vi "BiaxXsig process (16chan).vi"(0 "voltage data":sgl[](array[numeric]) format="%.2f", 3 "Numeric":i32=4, 7 "error in (no error)":errorcluster) -> (8 "signal to file (Volt)":sgl[](array[numeric]) format="%.2f", 9 "AUX8":dbl format="%.2f", 10 "AUX9":dbl format="%.2f", 11 "Hor LVDT":dbl format="%.2f", 12 "AUX7":dbl format="%.2f", 13 "AUX6":dbl format="%.2f", 14 "AUX5":dbl format="%.2f", 15 "error out":errorcluster, 16 "AUX12":dbl format="%.2f", 17 "AUX4":dbl format="%.2f", 18 "AUX11":dbl format="%.2f", 19 "AUX10":dbl format="%.2f", 20 "Hor Load":dbl format="%.2f", 21 "Vert Load":dbl format="%.2f", 23 "Ver LVDT":dbl format="%.2f", 24 "AUX1":dbl format="%.2f", 25 "AUX2":dbl format="%.2f", 27 "AUX3":dbl format="%.2f")   [LabVIEW 2013]
doc: "This vi accepts the raw voltage data from the following channels: \nCh 0 = Conf. Press. Amp. (0-5)\nCh 1 = Fluid Press. Amp (0-5)\nCh 2 = Temp. Amp (0-1.25 V)\nCh 3 = Displacement Transducer (-2.5 to +2.5 Volt)The data is acquired and processed one point at a time (a non-buffered acquisition). \nCh 4 = Load cell after amplification. 12600 lbsf/volt \n\nThe voltage data array contains the data that the example VI just retrieved from the buffer, one sample per channel. It is a one-dimensional array, indexed by channel.\n\nThe processed data array is returned to the example VI to be displayed.\n\nError in is a cluster that indicates if an error has occurred. If so, this VI does not try to process the data, it just returns the voltage data and error unchanged. If an error occurs in your data processing, you should set the following values in the error out cluster:\n\n (bool) status: TRUE.\n\n (i32) code: the error code associated with an error.\n A value of 0 means no error, a negative value is an error,\n and a positive value is a warning.\n\n (string) source: an indication of where the \n error occurred, usually the name of the VI."
panel:
  # "Sig. Eng. Units"
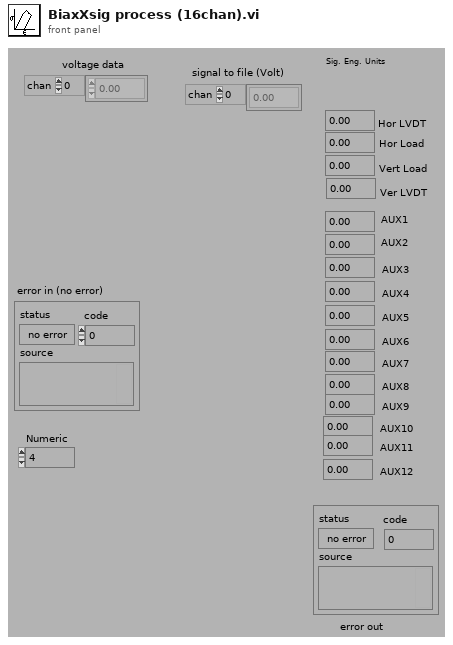
[diagram p1: front panel]
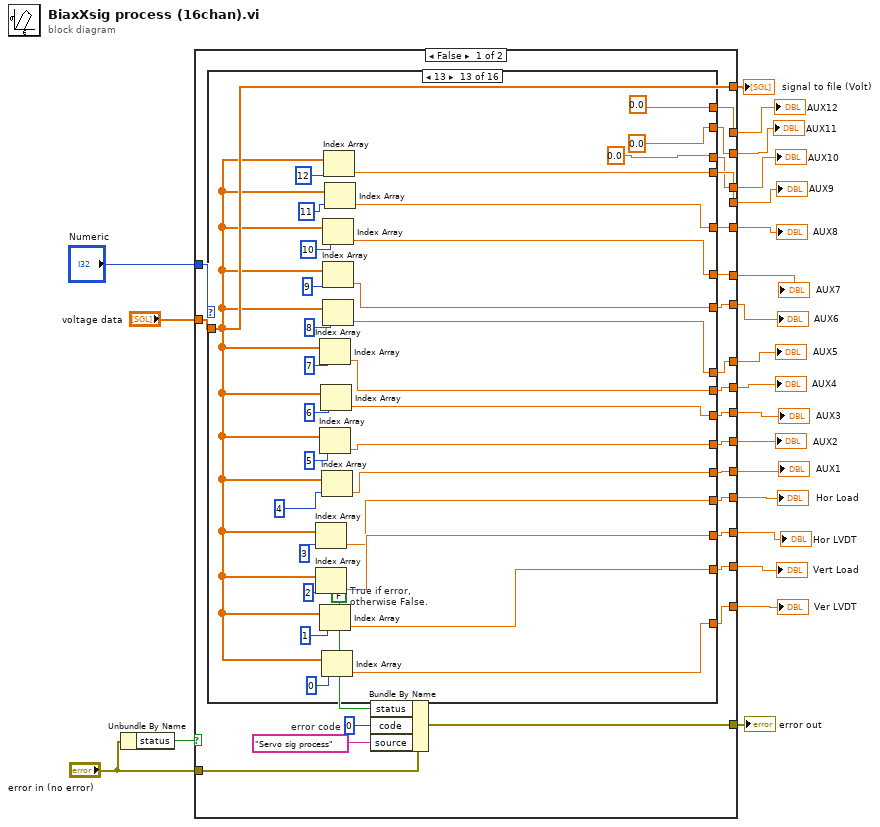
[diagram p0: block diagram]
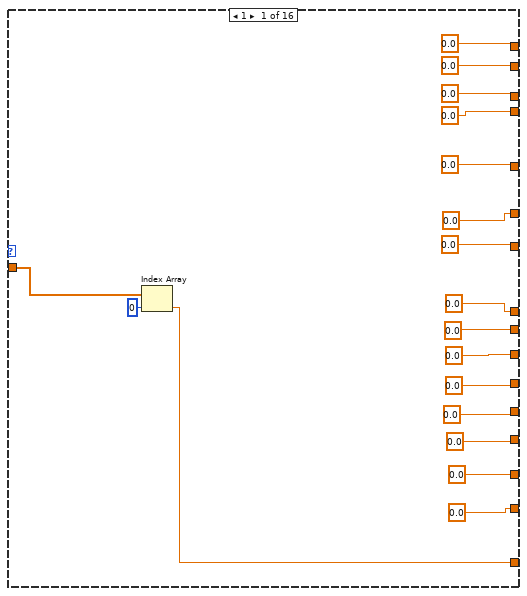
[diagram p2: hidden frame]
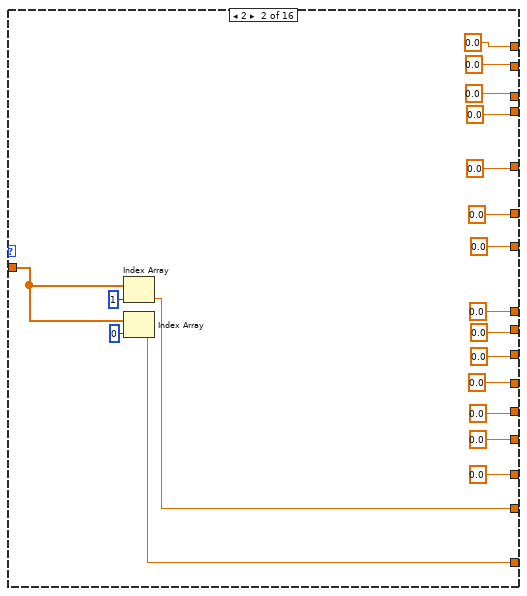
[diagram p3: hidden frame]
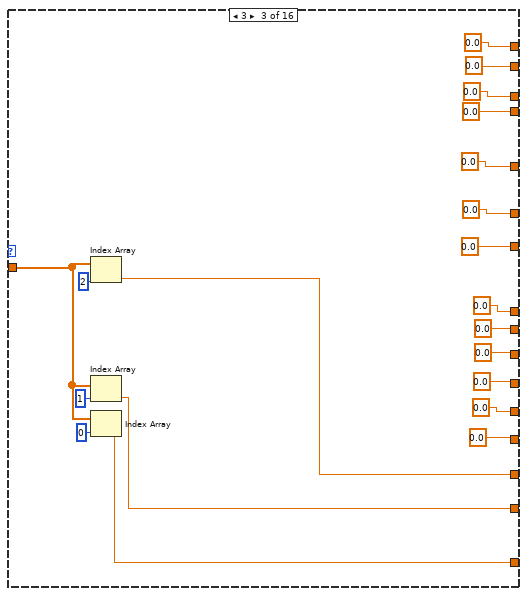
[diagram p4: hidden frame]
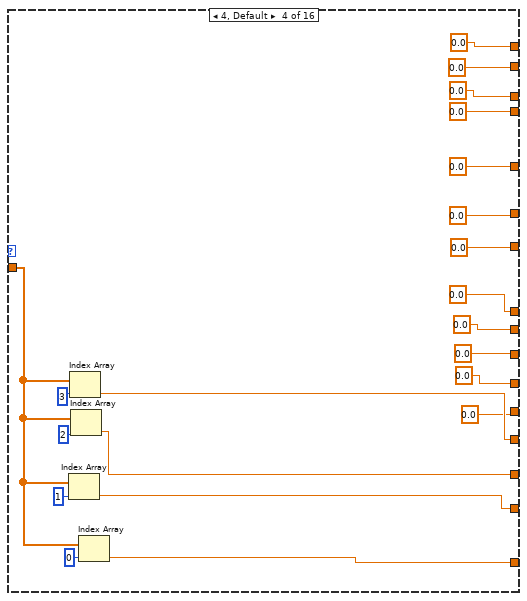
[diagram p5: hidden frame]
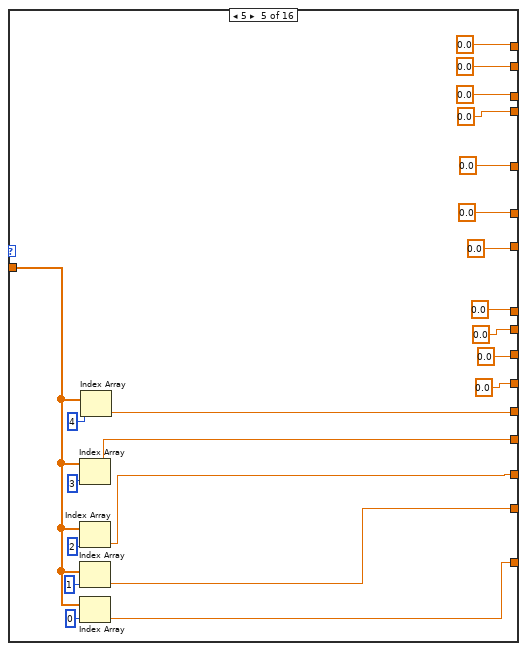
[diagram p6: hidden frame]
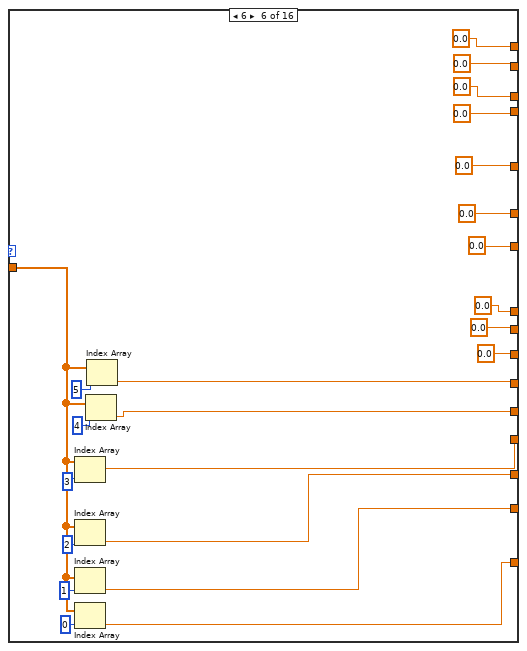
[diagram p7: hidden frame]
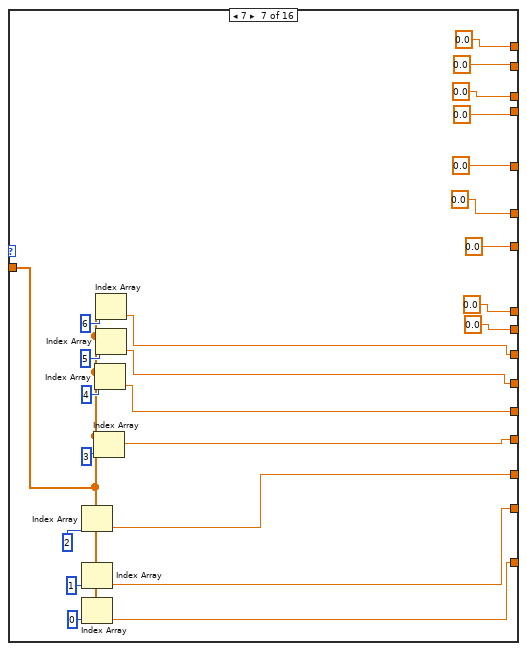
[diagram p8: hidden frame]
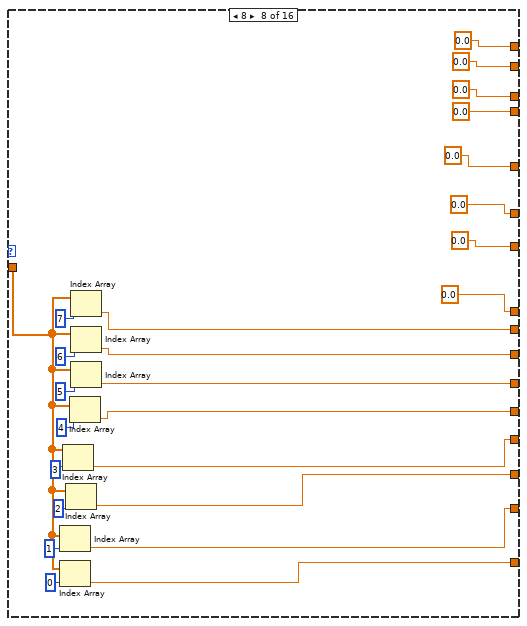
[diagram p9: hidden frame]
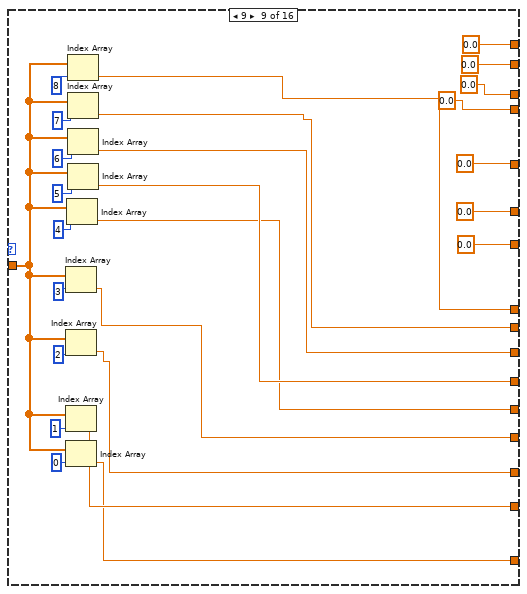
[diagram p10: hidden frame]
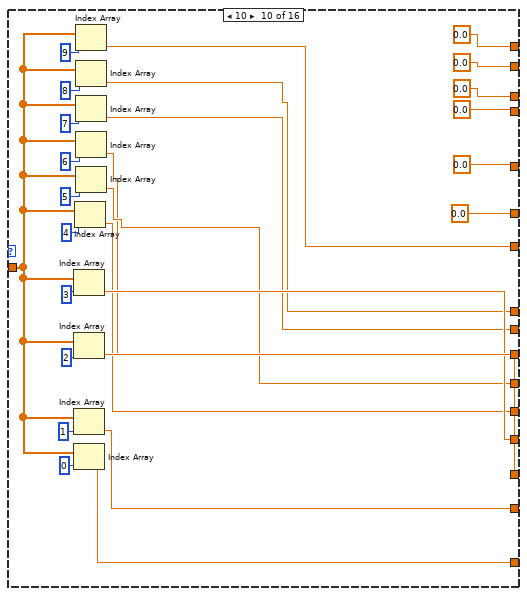
[diagram p11: hidden frame]
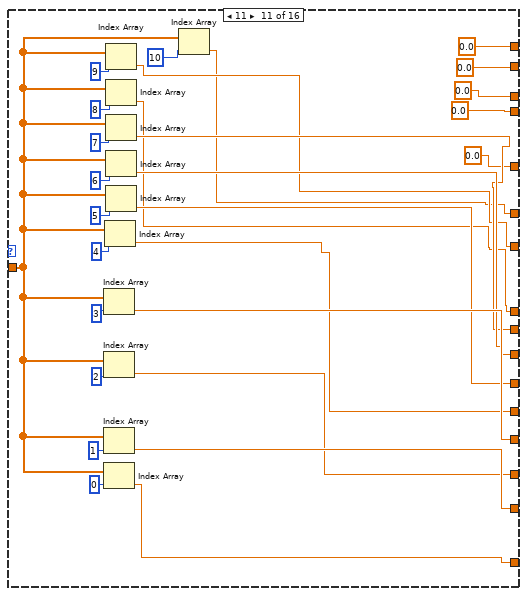
[diagram p12: hidden frame]
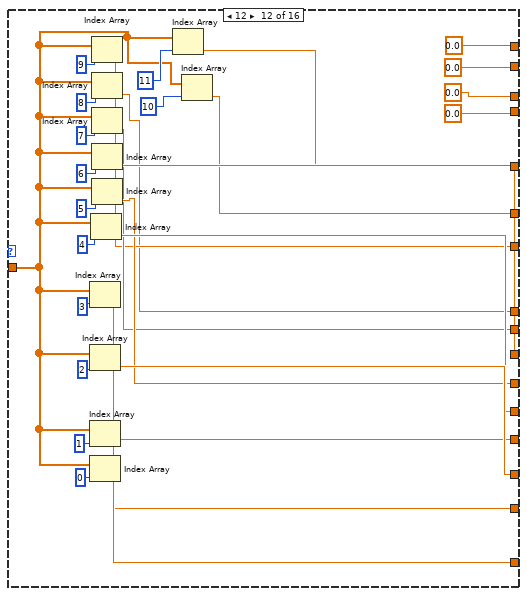
[diagram p13: hidden frame]
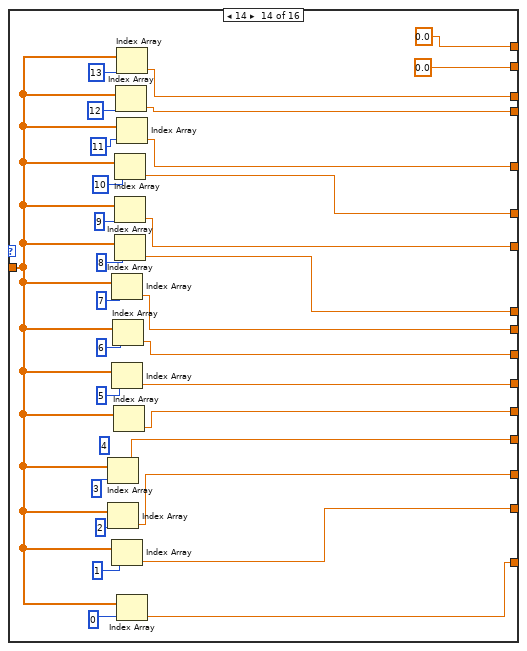
[diagram p14: hidden frame]
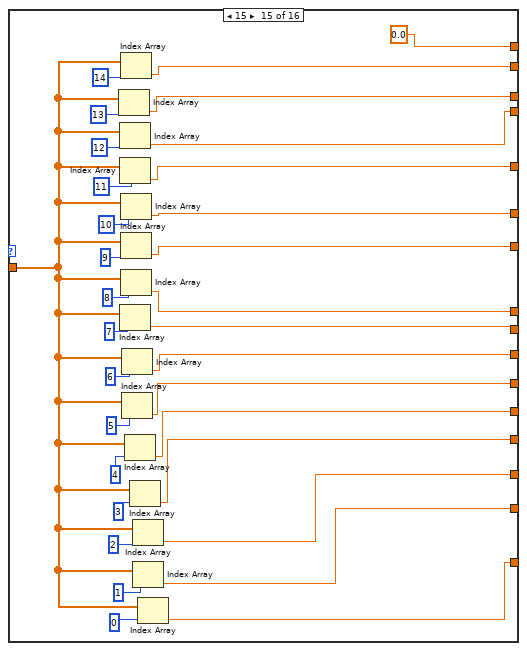
[diagram p15: hidden frame]
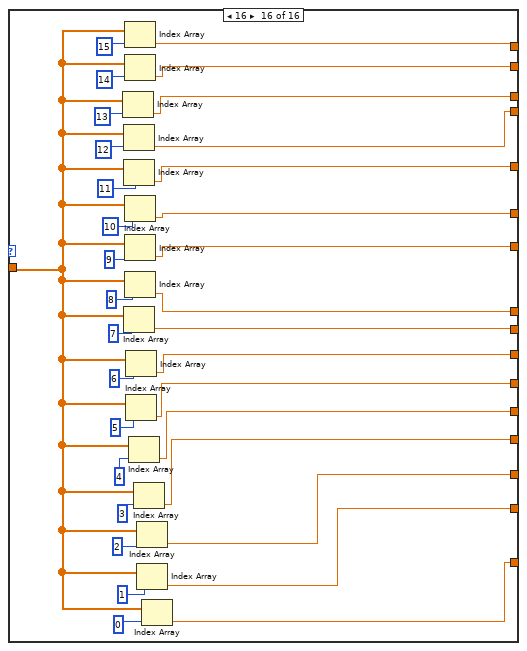
[diagram p16: hidden frame]
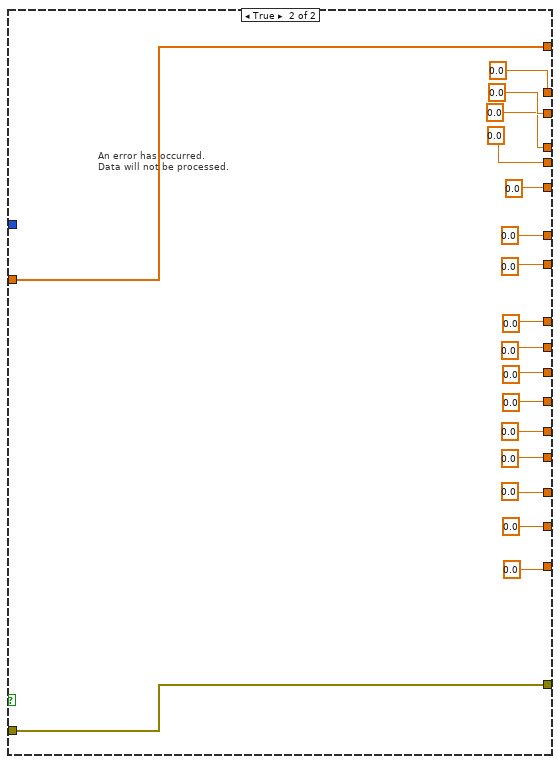
[diagram p17: hidden frame]
diagram:
  n1 = Unbundle By Name("error in (no error)") -> ("status"=w19:bool)
  n2 = case shown="False" w19 {
    tunnel: [w36 sgl 0.0] -> w15
    tunnel: "error in (no error)" -> [w41 w469]
    tunnel: [w45 w469] -> w22
    tunnel: "voltage data" -> [w40 w470]
    tunnel: [w40 w470] -> w20
    tunnel: "Numeric" -> [w39 _]
    tunnel: [w38 sgl 0.0] -> w10
    tunnel: [w37 sgl 0.0] -> w16
    tunnel: [w30 sgl 0.0] -> w14
    tunnel: [w35 sgl 0.0] -> w1
    tunnel: [w34 sgl 0.0] -> w13
    tunnel: [w33 sgl 0.0] -> w12
    tunnel: [w32 sgl 0.0] -> w11
    tunnel: [w25 sgl 0.0] -> w9
    tunnel: [w31 sgl 0.0] -> w8
    tunnel: [w24 sgl 0.0] -> w7
    tunnel: [w29 sgl 0.0] -> w6
    tunnel: [w28 sgl 0.0] -> w5
    tunnel: [w23 sgl 0.0] -> w4
    tunnel: [w27 sgl 0.0] -> w3
    tunnel: [w26 sgl 0.0] -> w2
    frame False {
      w44 = 0  # error code
      w42 = FALSE  # True if error, otherwise False.
      n3 = case shown="13" w39 {
        tunnel: w40 -> [w62 w80 w99 w119 w140 w162 w178 w209 w228 w251 w278 w315 w345 w372 w389 w439]
        tunnel: [sgl 0.0 sgl 0.0 sgl 0.0 sgl 0.0 sgl 0.0 sgl 0.0 sgl 0.0 w208 w222 w253 w280 w307 w337 w364 w397 w430] -> w38
        tunnel: [sgl 0.0 sgl 0.0 sgl 0.0 sgl 0.0 sgl 0.0 sgl 0.0 w179 w207 w223 w254 w281 w308 w338 w365 w398 w431] -> w37
        tunnel: [sgl 0.0 sgl 0.0 sgl 0.0 sgl 0.0 sgl 0.0 w161 w180 w206 w235 w255 w282 w309 w339 w366 w399 w432] -> w36
        tunnel: [sgl 0.0 sgl 0.0 w98 w116 w137 w158 w183 w205 w232 w258 w285 w312 w342 w369 w402 w435] -> w35
        tunnel: [sgl 0.0 w79 w97 w117 w136 w157 w184 w204 w231 w259 w286 w313 w343 w370 w403 w436] -> w34
        tunnel: [w61 w78 w96 w118 w135 w156 w185 w203 w230 w260 w287 w314 w344 w371 w404 w437] -> w33
        tunnel: [sgl 0.0 sgl 0.0 sgl 0.0 sgl 0.0 w139 w160 w181 w202 w234 w256 w283 w310 w340 w367 w400 w433] -> w32
        tunnel: [sgl 0.0 sgl 0.0 sgl 0.0 sgl 0.0 sgl 0.0 sgl 0.0 sgl 0.0 sgl 0.0 sgl 0.0 w252 w279 w306 w336 w362 w395 w429] -> w31
        tunnel: [sgl 0.0 sgl 0.0 sgl 0.0 sgl 0.0 sgl 0.0 sgl 0.0 sgl 0.0 sgl 0.0 sgl 0.0 sgl 0.0 sgl 0.0 w305 w335 w360 w393 w426] -> w29
        tunnel: [sgl 0.0 sgl 0.0 sgl 0.0 w115 w138 w159 w182 w201 w233 w257 w284 w311 w341 w368 w401 w434] -> w30
        tunnel: [sgl 0.0 sgl 0.0 sgl 0.0 sgl 0.0 sgl 0.0 sgl 0.0 sgl 0.0 sgl 0.0 sgl 0.0 sgl 0.0 sgl 0.0 sgl 0.0 w334 w359 w392 w425] -> w28
        tunnel: [sgl 0.0 sgl 0.0 sgl 0.0 sgl 0.0 sgl 0.0 sgl 0.0 sgl 0.0 sgl 0.0 sgl 0.0 sgl 0.0 sgl 0.0 sgl 0.0 sgl 0.0 sgl 0.0 sgl 0.0 w438] -> w23
        tunnel: [sgl 0.0 sgl 0.0 sgl 0.0 sgl 0.0 sgl 0.0 sgl 0.0 sgl 0.0 sgl 0.0 sgl 0.0 sgl 0.0 sgl 0.0 sgl 0.0 sgl 0.0 sgl 0.0 w388 w440] -> w27
        tunnel: [sgl 0.0 sgl 0.0 sgl 0.0 sgl 0.0 sgl 0.0 sgl 0.0 sgl 0.0 sgl 0.0 sgl 0.0 sgl 0.0 sgl 0.0 sgl 0.0 sgl 0.0 w358 w391 w424] -> w26
        tunnel: [sgl 0.0 sgl 0.0 sgl 0.0 sgl 0.0 sgl 0.0 sgl 0.0 sgl 0.0 sgl 0.0 w219 w244 w271 w299 w330 w363 w396 w428] -> w25
        tunnel: [sgl 0.0 sgl 0.0 sgl 0.0 sgl 0.0 sgl 0.0 sgl 0.0 sgl 0.0 sgl 0.0 sgl 0.0 sgl 0.0 w272 w300 w329 w361 w394 w427] -> w24
        frame 1 {
          n4 = Index Array(array=w62, index=0) -> (element=w61:sgl)
        }
        frame 2 {
          n5 = Index Array(array=w80, index=1) -> (element=w79:sgl)
          n6 = Index Array(array=w80, index=0) -> (element=w78:sgl)
        }
        frame 3 {
          n7 = Index Array(array=w99, index=2) -> (element=w98:sgl)
          n8 = Index Array(array=w99, index=1) -> (element=w97:sgl)
          n9 = Index Array(array=w99, index=0) -> (element=w96:sgl)
        }
        frame 4, Default {
          n10 = Index Array(array=w119, index=1) -> (element=w117:sgl)
          n11 = Index Array(array=w119, index=3) -> (element=w115:sgl)
          n12 = Index Array(array=w119, index=2) -> (element=w116:sgl)
          n13 = Index Array(array=w119, index=0) -> (element=w118:sgl)
        }
        frame 5 {
          n14 = Index Array(array=w140, index=3) -> (element=w138:sgl)
          n15 = Index Array(array=w140, index=2) -> (element=w137:sgl)
          n16 = Index Array(array=w140, index=1) -> (element=w136:sgl)
          n17 = Index Array(array=w140, index=0) -> (element=w135:sgl)
          n18 = Index Array(array=w140, index=4) -> (element=w139:sgl)
        }
        frame 6 {
          n19 = Index Array(array=w162, index=3) -> (element=w159:sgl)
          n20 = Index Array(array=w162, index=2) -> (element=w158:sgl)
          n21 = Index Array(array=w162, index=1) -> (element=w157:sgl)
          n22 = Index Array(array=w162, index=0) -> (element=w156:sgl)
          n23 = Index Array(array=w162, index=4) -> (element=w160:sgl)
          n24 = Index Array(array=w162, index=5) -> (element=w161:sgl)
        }
        frame 7 {
          n25 = Index Array(array=w178, index=2) -> (element=w183:sgl)
          n26 = Index Array(array=w178, index=1) -> (element=w184:sgl)
          n27 = Index Array(array=w178, index=0) -> (element=w185:sgl)
          n28 = Index Array(array=w178, index=3) -> (element=w182:sgl)
          n29 = Index Array(array=w178, index=4) -> (element=w181:sgl)
          n30 = Index Array(array=w178, index=6) -> (element=w179:sgl)
          n31 = Index Array(array=w178, index=5) -> (element=w180:sgl)
        }
        frame 8 {
          n32 = Index Array(array=w209, index=1) -> (element=w204:sgl)
          n33 = Index Array(array=w209, index=0) -> (element=w203:sgl)
          n34 = Index Array(array=w209, index=3) -> (element=w201:sgl)
          n35 = Index Array(array=w209, index=2) -> (element=w205:sgl)
          n36 = Index Array(array=w209, index=4) -> (element=w202:sgl)
          n37 = Index Array(array=w209, index=7) -> (element=w208:sgl)
          n38 = Index Array(array=w209, index=6) -> (element=w207:sgl)
          n39 = Index Array(array=w209, index=5) -> (element=w206:sgl)
        }
        frame 9 {
          n40 = Index Array(array=w228, index=3) -> (element=w233:sgl)
          n41 = Index Array(array=w228, index=2) -> (element=w232:sgl)
          n42 = Index Array(array=w228, index=1) -> (element=w231:sgl)
          n43 = Index Array(array=w228, index=0) -> (element=w230:sgl)
          n44 = Index Array(array=w228, index=4) -> (element=w234:sgl)
          n45 = Index Array(array=w228, index=8) -> (element=w219:sgl)
          n46 = Index Array(array=w228, index=7) -> (element=w222:sgl)
          n47 = Index Array(array=w228, index=6) -> (element=w223:sgl)
          n48 = Index Array(array=w228, index=5) -> (element=w235:sgl)
        }
        frame 10 {
          n49 = Index Array(array=w251, index=3) -> (element=w257:sgl)
          n50 = Index Array(array=w251, index=2) -> (element=w258:sgl)
          n51 = Index Array(array=w251, index=1) -> (element=w259:sgl)
          n52 = Index Array(array=w251, index=0) -> (element=w260:sgl)
          n53 = Index Array(array=w251, index=4) -> (element=w256:sgl)
          n54 = Index Array(array=w251, index=9) -> (element=w252:sgl)
          n55 = Index Array(array=w251, index=8) -> (element=w244:sgl)
          n56 = Index Array(array=w251, index=7) -> (element=w253:sgl)
          n57 = Index Array(array=w251, index=6) -> (element=w254:sgl)
          n58 = Index Array(array=w251, index=5) -> (element=w255:sgl)
        }
        frame 11 {
          n59 = Index Array(array=w278, index=3) -> (element=w284:sgl)
          n60 = Index Array(array=w278, index=2) -> (element=w285:sgl)
          n61 = Index Array(array=w278, index=1) -> (element=w286:sgl)
          n62 = Index Array(array=w278, index=0) -> (element=w287:sgl)
          n63 = Index Array(array=w278, index=4) -> (element=w283:sgl)
          n64 = Index Array(array=w278, index=9) -> (element=w279:sgl)
          n65 = Index Array(array=w278, index=8) -> (element=w271:sgl)
          n66 = Index Array(array=w278, index=7) -> (element=w280:sgl)
          n67 = Index Array(array=w278, index=6) -> (element=w281:sgl)
          n68 = Index Array(array=w278, index=5) -> (element=w282:sgl)
          n69 = Index Array(array=w278, index=10) -> (element=w272:sgl)
        }
        frame 12 {
          n70 = Index Array(array=w315, index=3) -> (element=w311:sgl)
          n71 = Index Array(array=w315, index=2) -> (element=w312:sgl)
          n72 = Index Array(array=w315, index=1) -> (element=w313:sgl)
          n73 = Index Array(array=w315, index=0) -> (element=w314:sgl)
          n74 = Index Array(array=w315, index=4) -> (element=w310:sgl)
          n75 = Index Array(array=w315, index=9) -> (element=w306:sgl)
          n76 = Index Array(array=w315, index=8) -> (element=w299:sgl)
          n77 = Index Array(array=w315, index=7) -> (element=w307:sgl)
          n78 = Index Array(array=w315, index=6) -> (element=w308:sgl)
          n79 = Index Array(array=w315, index=5) -> (element=w309:sgl)
          n80 = Index Array(array=w315, index=11) -> (element=w305:sgl)
          n81 = Index Array(array=w315, index=10) -> (element=w300:sgl)
        }
        frame 13 {
          n82 = Index Array(array=w345, index=3) -> (element=w341:sgl)
          n83 = Index Array(array=w345, index=2) -> (element=w342:sgl)
          n84 = Index Array(array=w345, index=7) -> (element=w337:sgl)
          n85 = Index Array(array=w345, index=5) -> (element=w339:sgl)
          n86 = Index Array(array=w345, index=1) -> (element=w343:sgl)
          n87 = Index Array(array=w345, index=6) -> (element=w338:sgl)
          n88 = Index Array(array=w345, index=4) -> (element=w340:sgl)
          n89 = Index Array(array=w345, index=0) -> (element=w344:sgl)
          n90 = Index Array(array=w345, index=10) -> (element=w329:sgl)
          n91 = Index Array(array=w345, index=9) -> (element=w336:sgl)
          n92 = Index Array(array=w345, index=8) -> (element=w330:sgl)
          n93 = Index Array(array=w345, index=12) -> (element=w334:sgl)
          n94 = Index Array(array=w345, index=11) -> (element=w335:sgl)
        }
        frame 14 {
          (unwired) 4
          n95 = Index Array(array=w372, index=3) -> (element=w368:sgl)
          n96 = Index Array(array=w372, index=2) -> (element=w369:sgl)
          n97 = Index Array(array=w372, index=7) -> (element=w364:sgl)
          n98 = Index Array(array=w372, index=5) -> (element=w366:sgl)
          n99 = Index Array(array=w372, index=1) -> (element=w370:sgl)
          n100 = Index Array(array=w372, index=6) -> (element=w365:sgl)
          n101 = Index Array(array=w372) -> (element=w367:sgl)  [unwired: 1 in]
          n102 = Index Array(array=w372, index=10) -> (element=w361:sgl)
          n103 = Index Array(array=w372, index=9) -> (element=w362:sgl)
          n104 = Index Array(array=w372, index=8) -> (element=w363:sgl)
          n105 = Index Array(array=w372, index=12) -> (element=w359:sgl)
          n106 = Index Array(array=w372, index=13) -> (element=w358:sgl)
          n107 = Index Array(array=w372, index=11) -> (element=w360:sgl)
          n108 = Index Array(array=w372, index=0) -> (element=w371:sgl)
        }
        frame 15 {
          n109 = Index Array(array=w389, index=13) -> (element=w391:sgl)
          n110 = Index Array(array=w389, index=12) -> (element=w392:sgl)
          n111 = Index Array(array=w389, index=11) -> (element=w393:sgl)
          n112 = Index Array(array=w389, index=7) -> (element=w397:sgl)
          n113 = Index Array(array=w389, index=14) -> (element=w388:sgl)
          n114 = Index Array(array=w389, index=10) -> (element=w394:sgl)
          n115 = Index Array(array=w389, index=9) -> (element=w395:sgl)
          n116 = Index Array(array=w389, index=8) -> (element=w396:sgl)
          n117 = Index Array(array=w389, index=6) -> (element=w398:sgl)
          n118 = Index Array(array=w389, index=5) -> (element=w399:sgl)
          n119 = Index Array(array=w389, index=4) -> (element=w400:sgl)
          n120 = Index Array(array=w389, index=3) -> (element=w401:sgl)
          n121 = Index Array(array=w389, index=2) -> (element=w402:sgl)
          n122 = Index Array(array=w389, index=1) -> (element=w403:sgl)
          n123 = Index Array(array=w389, index=0) -> (element=w404:sgl)
        }
        frame 16 {
          n124 = Index Array(array=w439, index=13) -> (element=w424:sgl)
          n125 = Index Array(array=w439, index=12) -> (element=w425:sgl)
          n126 = Index Array(array=w439, index=11) -> (element=w426:sgl)
          n127 = Index Array(array=w439, index=7) -> (element=w430:sgl)
          n128 = Index Array(array=w439, index=15) -> (element=w438:sgl)
          n129 = Index Array(array=w439, index=14) -> (element=w440:sgl)
          n130 = Index Array(array=w439, index=10) -> (element=w427:sgl)
          n131 = Index Array(array=w439, index=9) -> (element=w429:sgl)
          n132 = Index Array(array=w439, index=8) -> (element=w428:sgl)
          n133 = Index Array(array=w439, index=6) -> (element=w431:sgl)
          n134 = Index Array(array=w439, index=5) -> (element=w432:sgl)
          n135 = Index Array(array=w439, index=4) -> (element=w433:sgl)
          n136 = Index Array(array=w439, index=3) -> (element=w434:sgl)
          n137 = Index Array(array=w439, index=2) -> (element=w435:sgl)
          n138 = Index Array(array=w439, index=1) -> (element=w436:sgl)
          n139 = Index Array(array=w439, index=0) -> (element=w437:sgl)
        }
      }
      n140 = Bundle By Name(cluster=w41, "status"=w42, "code"=w44, "source"="Servo sig process") -> (w45:errorcluster)
    }
    frame True {
      # "An error has occurred.\nData will not be processed."
    }
  }
  "signal to file (Volt)" <- w20
  "error out" <- w22
  "Vert Load" <- w13
  "Ver LVDT" <- w12
  "Hor Load" <- w14
  "AUX1" <- w11
  "AUX2" <- w15
  "AUX3" <- w16
  "AUX4" <- w10
  "AUX5" <- w9
  "AUX6" <- w8
  "AUX7" <- w7
  "AUX8" <- w6
  "AUX9" <- w5
  "AUX12" <- w4
  "AUX10" <- w2
  "AUX11" <- w3
  "Hor LVDT" <- w1
